vi "main2.vi"() -> ()   [LabVIEW 2018]
uses:
  <vilib>/httpClient/LabVIEWHTTPClient.lvlib
panel:
  in  "error in (no error)":errorcluster
  in  "value":string
  in  "header":string(combo)="User-Agent"
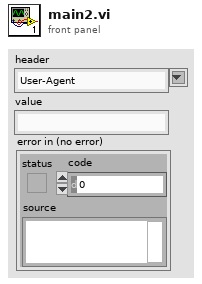
[diagram p1: front panel]
types:
  T1 = typedef "LabVIEWHTTPClient.lvlib/ClientHandle.ctl" = refnum<k1>
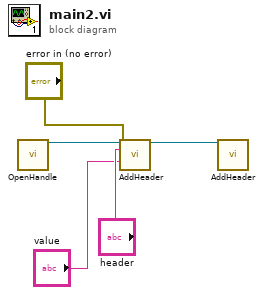
[diagram p0: block diagram]
diagram:
  n1 = call <vilib>:"OpenHandle.vi"() -> ("client handle out"=w5:T1)  [unwired: 14 in, 1 out]
  n2 = call <vilib>:"AddHeader.vi"("client handle"=w5, "header"="header", "value"="value", "error in (no error)"="error in (no error)") -> ("client handle out"=w4:T1)  [unwired: 10 in, 1 out]
  n3 = call <vilib>:"AddHeader.vi"("client handle"=w4) -> ()  [unwired: 13 in, 2 out]
